vi "Solve for Reachable Velocity.vi"(1 "Max Acceleration":dbl, 2 "Max Velocity":dbl, 3 "Angular Displacement":dbl) -> (0 "Reachable Velocity":dbl)   [LabVIEW 2015]
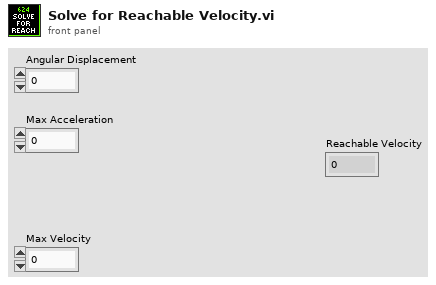
[diagram p1: front panel]
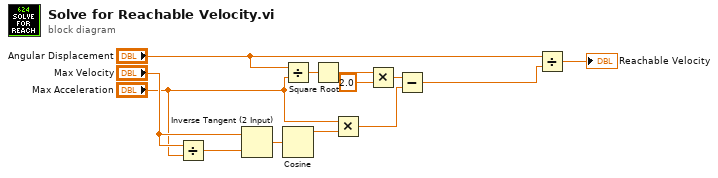
[diagram p0: block diagram]
diagram:
  n1 = Divide(x="Max Velocity", y="Max Acceleration") -> (x/y=w1:dbl)
  n2 = Inverse Tangent (2 Input)(1:w1, 2:"Max Velocity") -> (0:w8:dbl)
  n3 = Divide(x="Angular Displacement", y="Max Acceleration") -> (x/y=w11:dbl)
  n4 = Cosine(x=w8) -> (cos(x)=w7:dbl)
  n5 = Square Root(x=w11) -> (sqrt(x)=w10:dbl)
  n6 = Multiply(x="Max Acceleration", y=w7) -> (x*y=w6:dbl)
  n7 = Multiply(x=w10, y=2.0) -> (x*y=w9:dbl)
  n8 = Subtract(x=w9, y=w6) -> (x-y=w5:dbl)
  n9 = Divide(x="Angular Displacement", y=w5) -> (x/y=→"Reachable Velocity":dbl)
